vi "validate.vi"(8 "error in":errorcluster, 11 "dds configuration in":refnum<class "dds configuration.lvclass">) -> (0 "error out":errorcluster, 3 "dds configuration out":refnum<class "dds configuration.lvclass">)   [LabVIEW 2020, in "DDS configuration.lvclass"]
doc: "This function performs validation of the configuration. This function should be safe to call at any point and should not rely on anything in the runtime environment."
uses:
  dds configuration.lvclass
  <vilib>/NI/Tag Bus Module Framework/module configuration/TBM module configuration.lvclass
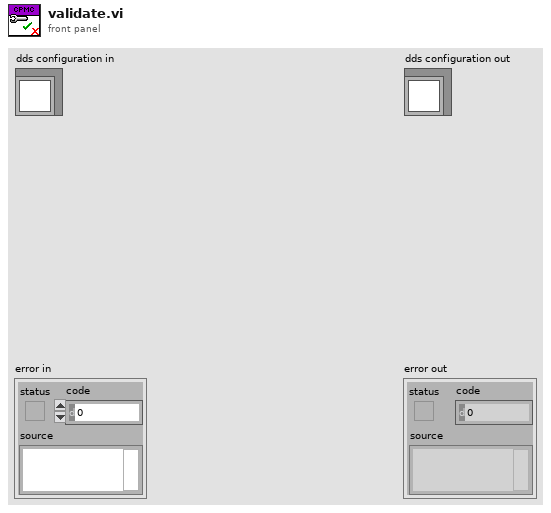
[diagram p1: front panel]
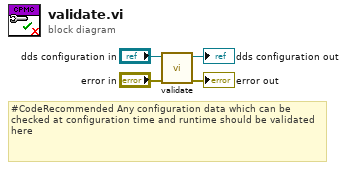
[diagram p0: block diagram]
diagram:
  # "#CodeRecommended Any configuration data which can be checked at configuration time and runtime should be validated here"
  n1 = call-parent "validate.vi"("error in"="error in", "configuration in"="dds configuration in") -> ("error out"=→"error out":errorcluster, "configuration out"=→"dds configuration out":refnum<class "dds configuration.lvclass">)  [unwired: 8 in]
